vi "加标回收调试界面.vi"() -> ()   [LabVIEW 2016, in "质控单元V1.lvlib"]
uses:
  <vilib>/Utility/miscctls.llb/LVPointTypeDef.ctl
  <vilib>/Utility/miscctls.llb/LVPositionTypeDef.ctl
panel:
  in  "关闭":bool
  in  "请选择模块":T1(radio)=enum."氨氮"
  in  "关于":bool
  in  "Tab Control 4":enum32{"参数"}(tab)
  out "加标体积":string
  out "告警状态":string
  out "液位状态":string
  out "运行状态":string
  out "通讯状态":bool caption="状态"
  in  "Tab Control 3":enum32{"参数设置"}(tab)
  out "Y3":bool
  out "Y1":bool
  out "Y0":bool
  out "X1":bool
  out "X0":bool
  out "脉冲数":i32
  out "频率":i32
  in  "定时刷新":bool
  in  "流程参数读取":bool
  in  "流程参数写入":bool
  out "排液时间":sgl format="%.2f"
  out "搅拌时间":sgl format="%.2f"
  out "进样时间":sgl format="%.2f"
  out "润洗进样时间2":sgl format="%.2f"
  out "润洗排液时间2":sgl format="%.2f"
  out "润洗排液时间1":sgl format="%.2f"
  out "润洗进样时间1":sgl format="%.2f"
  in  "加标体积读取":bool
  in  "加标体积写入":bool
  in  "B":sgl
  in  "K":sgl
  in  "加标体积(mL)":sgl
  in  "注射泵系数读取":bool
  in  "注射泵系数写入":bool
  in  "Tab Control 2":enum32{"参数"}(tab)
  in  "启动水样润洗流程":bool
  in  "启动进样流程":bool
  in  "启动加标流程":bool
  in  "启动排液流程":bool
  in  "停止所有流程":bool
  in  "组合操作进水样":T2
  in  "清除告警":bool
  in  "启动搅拌流程":bool
  in  "加标":bool
  in  "注射泵注入量":sgl=0.1 min=0 max=1000 format="%#.6f mL"
  in  "组合操作排废液":T2
  in  "组合操作进空气":T2
  in  "组合操作慢速到液位":T2
  in  "组合操作进样调速":T2
  # "仪器状态"
  # "(默认30S)"
  # "柱塞泵泵系数"
  # "(默认50S)"
  # "(默认140S)"
  # "(默认500S)"
  # "(默认500S)"
  # "IO状态"
  # "(默认60S)"
  # "(默认140S)"
  # "组合步骤"
  # "测试流程"
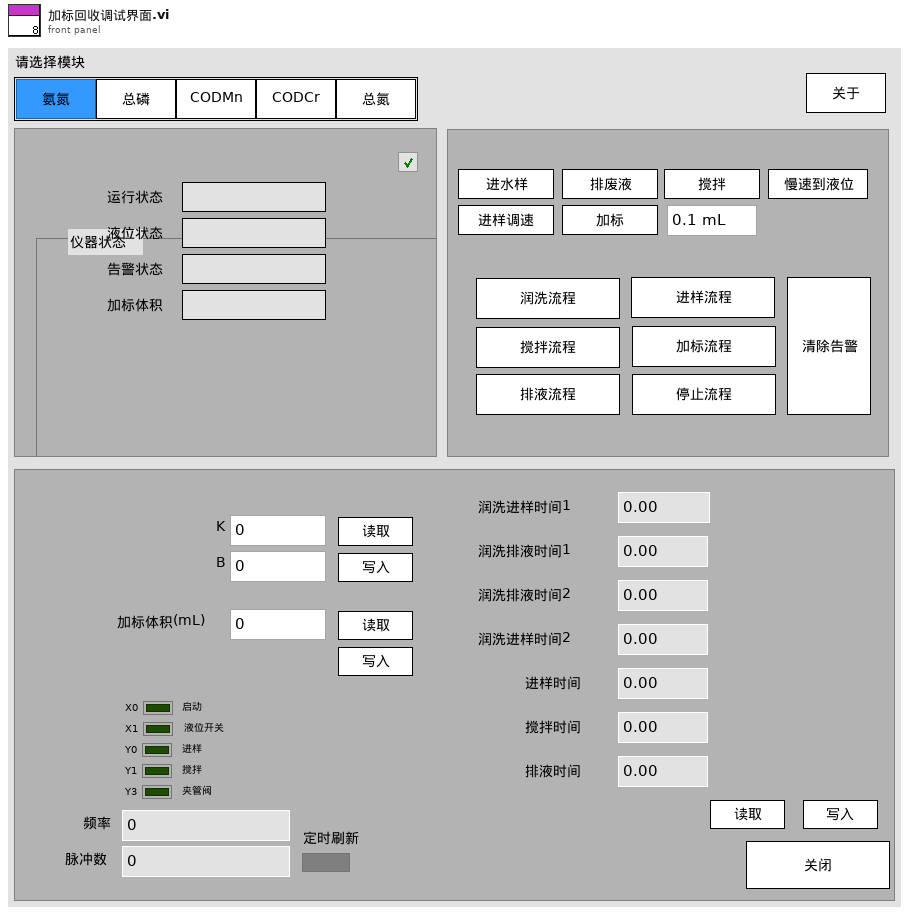
[diagram p1: front panel]
types:
  T1 = enum32{"未选择", "氨氮", "总磷", "CODMn", "CODCr", "总氮"}
  T2 = typedef "质控单元V1.lvlib/布尔控件.ctl" = bool
  T3 = typedef "LVPositionTypeDef.ctl" = cluster{"Left":i32, "Top":i32}
  T4 = typedef "LVPointTypeDef.ctl" = cluster{"Horizontal":i16, "Vertical":i16}
  T5 = typedef "质控单元V1.lvlib/质控slave id.ctl" = enum16{"null", "氨氮", "总磷", "CODMn", "CODCr", "总氮"}
  T6 = typedef "质控单元V1.lvlib/质控流程控制.ctl" = enum16{"待机", "润洗", "进样", "加标", "排液", "搅拌"}
  T7 = typedef "质控单元V1.lvlib/质控仪器状态显示.ctl" = cluster{"运行模式":string, "运行状态":string, "液位状态":string, "告警状态":string, "加标体积":string}
  T8 = cluster{"X0":bool, "X1":bool, "Y0":bool, "Y1":bool, "Y2":bool, "Y3":bool, "频率":i32, "脉冲数":i32}
  T9 = cluster{"润洗进样时间":sgl, "润洗排液时间1":sgl, "润洗排液时间2":sgl, "润洗超时时间":sgl, "进样超时时间":sgl, "搅拌时间":sgl, "排液时间":sgl}
  T10 = cluster{"润洗进样时间1":sgl, "润洗排液时间1":sgl, "润洗排液时间2":sgl, "润洗进样时间2":sgl, "进样时间":sgl, "搅拌时间":sgl, "排液时间":sgl}
  T11 = typedef "LVRectTypeDef.ctl" = cluster{"Left":i16, "Top":i16, "Right":i16, "Bottom":i16}
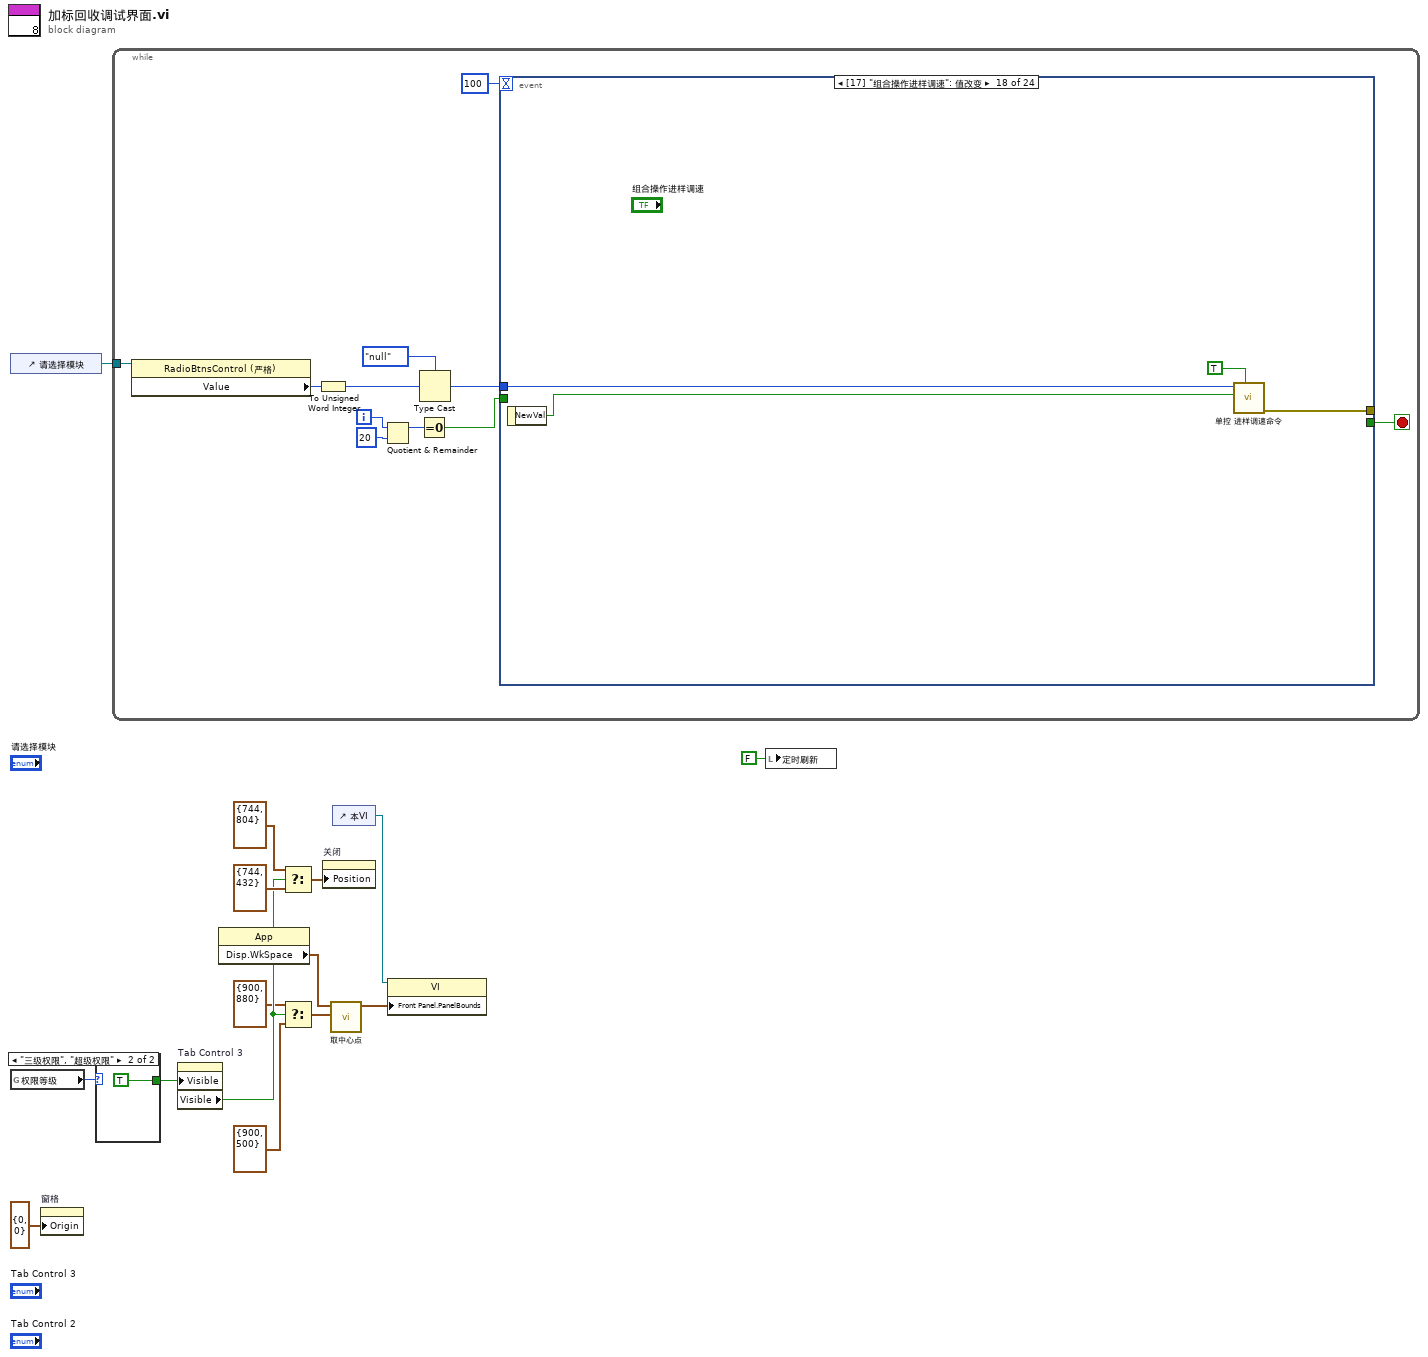
[diagram p0: block diagram]
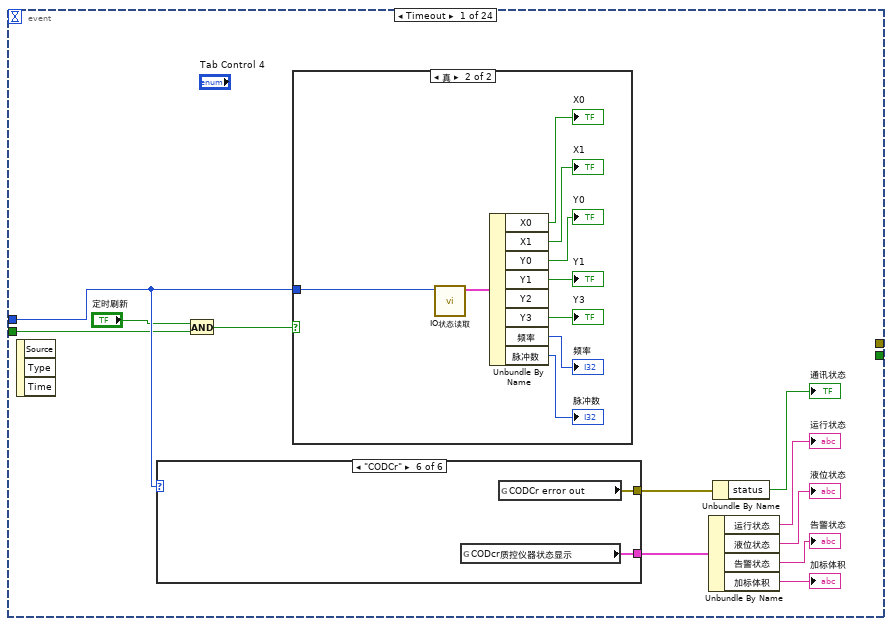
[diagram p3: hidden frame]
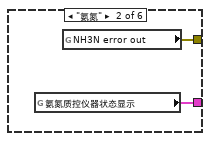
[diagram p6: hidden frame]
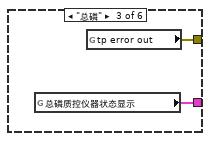
[diagram p7: hidden frame]
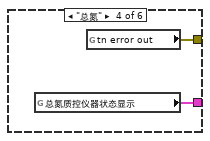
[diagram p8: hidden frame]
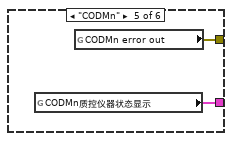
[diagram p9: hidden frame]
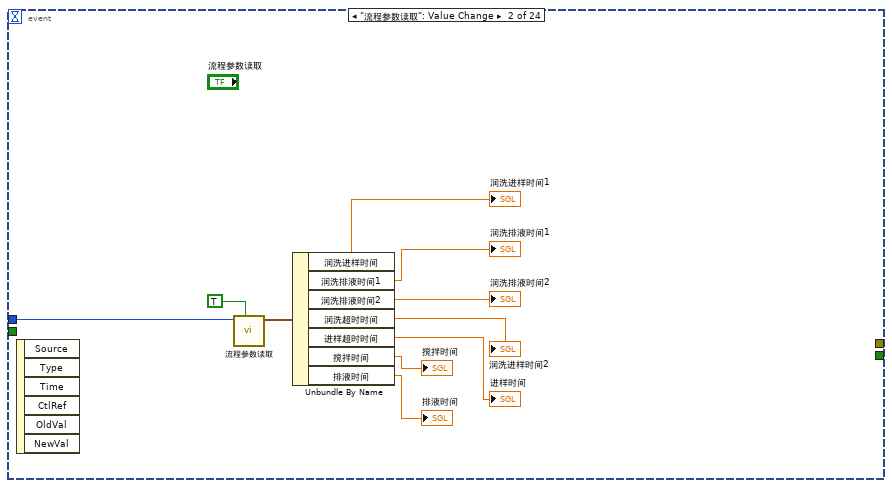
[diagram p10: hidden frame]
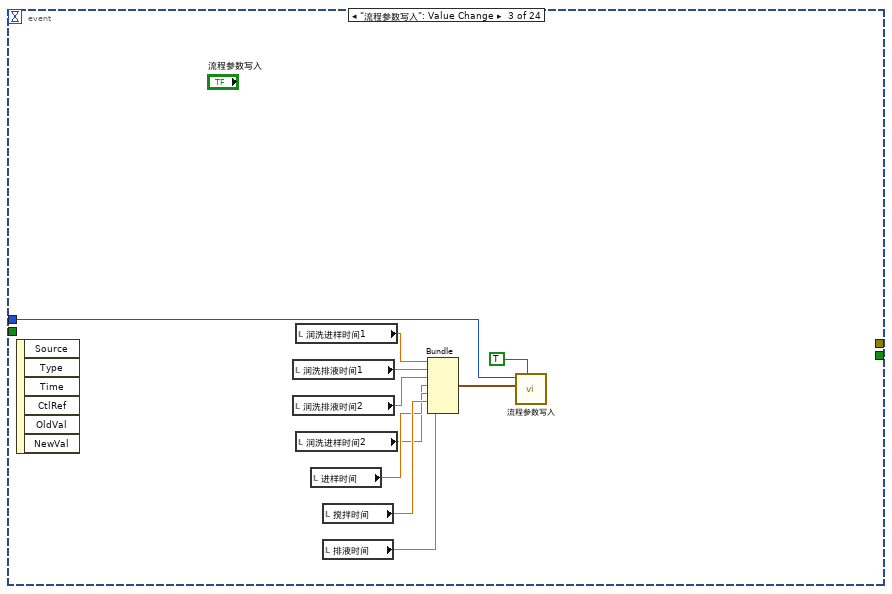
[diagram p11: hidden frame]
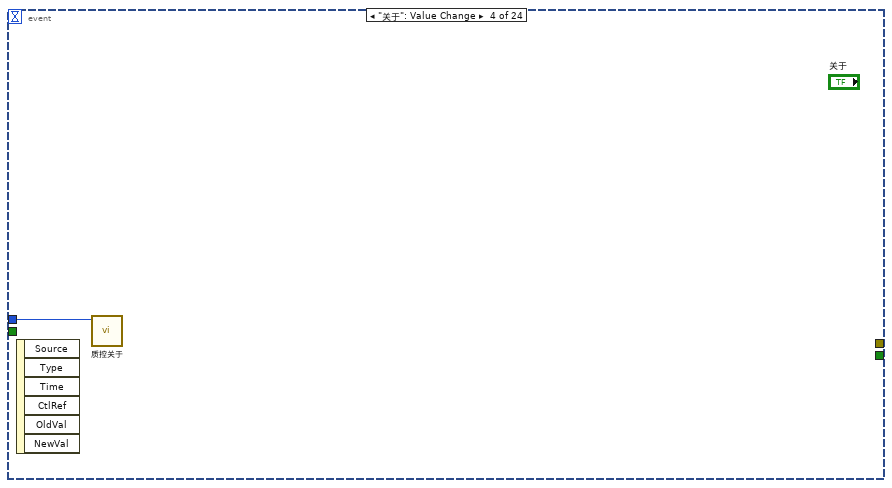
[diagram p12: hidden frame]
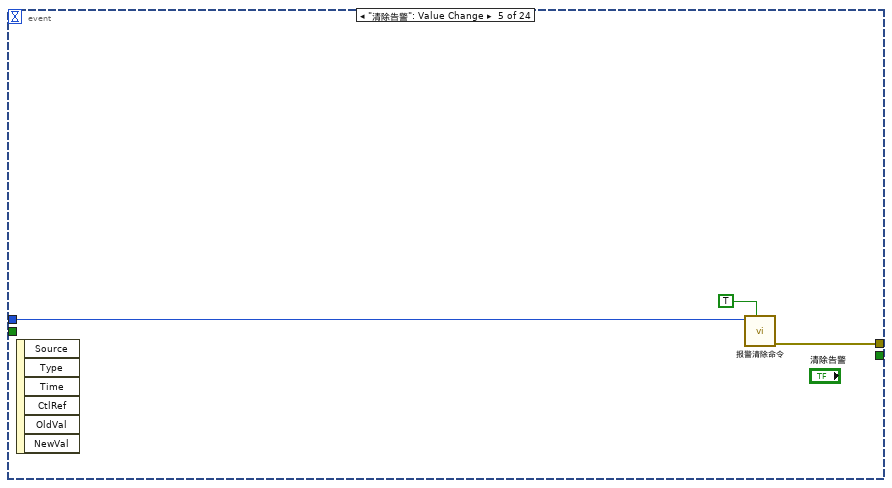
[diagram p13: hidden frame]
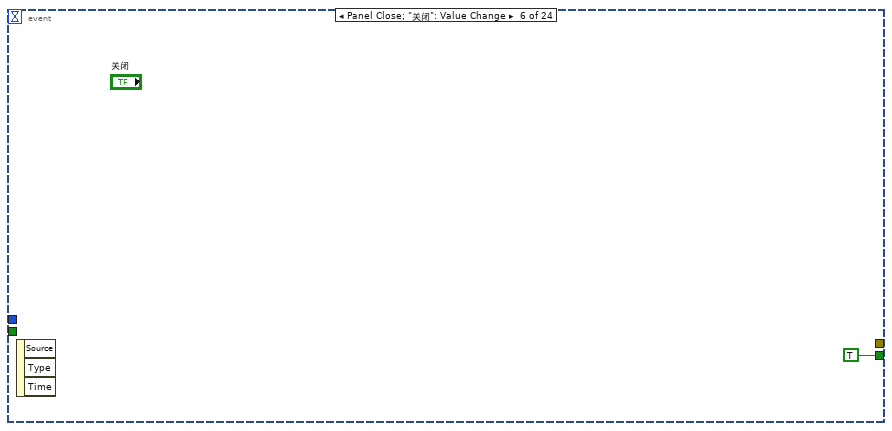
[diagram p14: hidden frame]
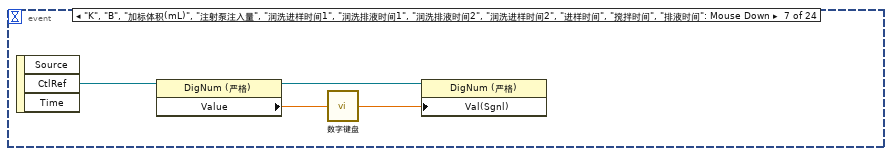
[diagram p15: hidden frame]
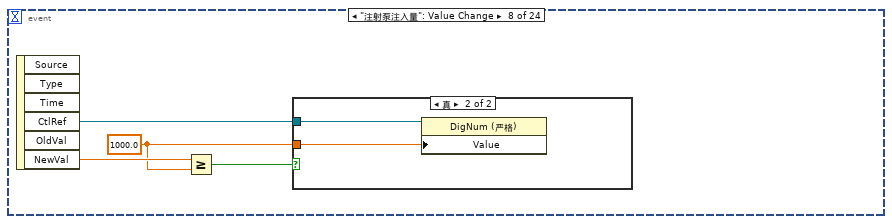
[diagram p16: hidden frame]
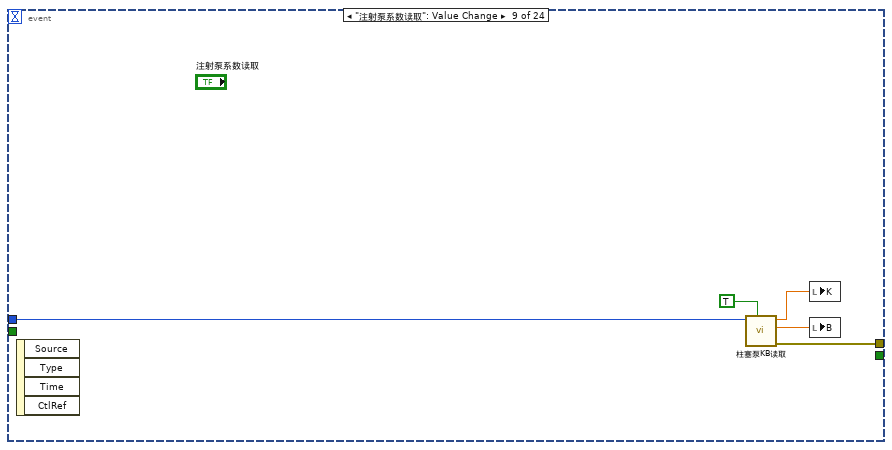
[diagram p18: hidden frame]
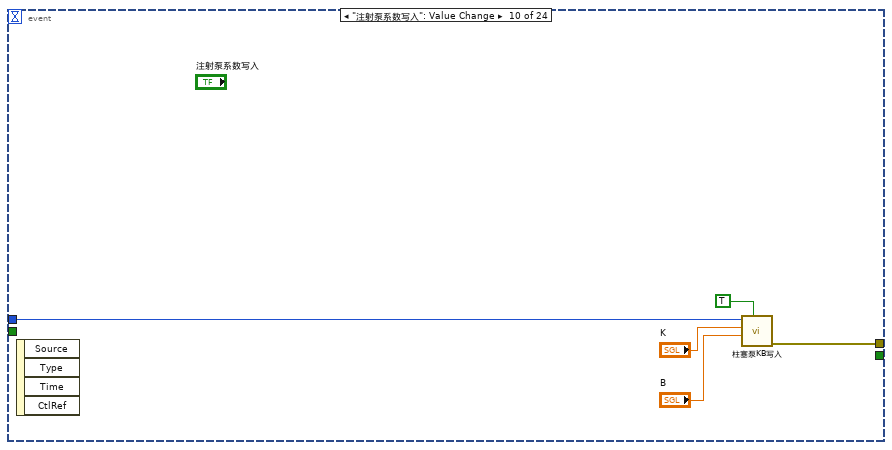
[diagram p19: hidden frame]
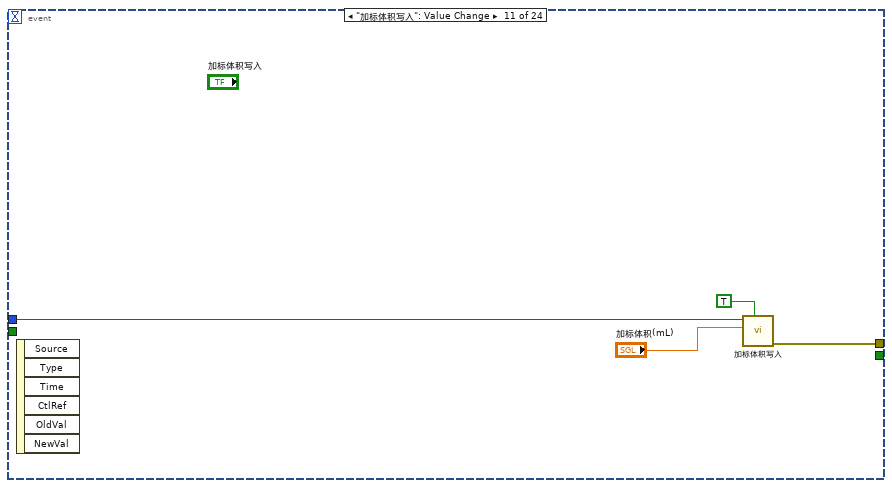
[diagram p20: hidden frame]
diagram:
  n1 = control-ref of="请选择模块"() -> (w14:refnum<vi>)
  n2 = global read "ZK非断电保存全局变量.vi" "权限等级"() -> (w3:enum16{"一级权限", "二级权限", "三级权限", "超级权限"})
  n3 = property on="窗格" class="Pane"("Origin"=T4 {"Horizontal"=0, "Vertical"=0} ("原点")) -> ()  [unwired: 2 in, 2 out]
  n4 = case shown="\"三级权限\", \"超级权限\"" w3 {
    tunnel: [_ TRUE] -> w2
    frame "一级权限", Default {
    }
    frame "三级权限", "超级权限" {
    }
  }
  n5 = while {
    tunnel: w14 -> [w25]
    i -> [w20]
    stop <- w27 stop-if-true
    n6 = property class="RadioBtnsControl (严格)"(reference=w25) -> ("Value"=w22:T1)  [unwired: 1 in, 2 out]
    n7 = To Unsigned Word Integer(number=w22) -> (unsigned 16bit integer=w21:u16)
    n8 = Quotient & Remainder(x=w20, y=20) -> (x-y*floor(x/y)=w18:i32)  [unwired: 1 out]
    n9 = Equal To 0?(x=w18) -> (x = 0?=w17:bool)
    n10 = Type Cast(type=质控slave_id."null" ("请选择模块"), x=w21) -> (*(type *) &x=w23:T5)
    n11 = event shown="[17] \"组合操作进样调速\": 值改变" {
      selector: _ -> [_ _ _ _ _ _ _ _ _ _ _ _ _ _ _ _ _ _ _ _ _ _ _ _]
      dyn-events: _ -> [_ _ _ _ _ _ _ _ _ _ _ _ _ _ _ _ _ _ _ _ _ _ _ _]
      timeout: 100 -> [_ _ _ _ _ _ _ _ _ _ _ _ _ _ _ _ _ _ _ _ _ _ _ _]
      tunnel: [_ _ _ _ _ TRUE _ _ _ _ _ _ _ _ _ _ _ _ _ _ _ _ _ _] -> w27
      tunnel: [_ _ _ _ w81 _ _ _ w95 w102 w106 w110 w113 w120 w124 w128 w132 w136 w140 w144 w148 w152 w155 w159] -> _
      tunnel: w23 -> [w31 w67 w77 w78 w79 _ _ _ w93 w100 w103 w107 w112 w118 w122 w126 w130 w134 w138 w141 w145 w149 w153 w157]
      tunnel: w17 -> [w29 _ _ _ _ _ _ _ _ _ _ _ _ _ _ _ _ _ _ _ _ _ _ _]
      event Timeout {
        n12 = event-data() -> ()  [unwired: 1 in, 3 out]
        n13 = case shown="\"CODCr\"" w31 {
          tunnel: [_ w49 w51 w53 w55 w57] -> w38
          tunnel: [_ w48 w50 w52 w54 w56] -> w33
          frame "null", Default {
          }
          frame "氨氮" {
            n14 = global read "ZK非断电保存全局变量.vi" "氨氮质控仪器状态显示"() -> (w49:T7)
            n15 = global read "ZK非断电保存全局变量.vi" "NH3N error out"() -> (w48:errorcluster)
          }
          frame "总磷" {
            n16 = global read "ZK非断电保存全局变量.vi" "总磷质控仪器状态显示"() -> (w51:T7)
            n17 = global read "ZK非断电保存全局变量.vi" "tp error out"() -> (w50:errorcluster)
          }
          frame "总氮" {
            n18 = global read "ZK非断电保存全局变量.vi" "总氮质控仪器状态显示"() -> (w53:T7)
            n19 = global read "ZK非断电保存全局变量.vi" "tn error out"() -> (w52:errorcluster)
          }
          frame "CODMn" {
            n20 = global read "ZK非断电保存全局变量.vi" "CODMn质控仪器状态显示"() -> (w55:T7)
            n21 = global read "ZK非断电保存全局变量.vi" "CODMn error out"() -> (w54:errorcluster)
          }
          frame "CODCr" {
            n22 = global read "ZK非断电保存全局变量.vi" "CODcr质控仪器状态显示"() -> (w57:T7)
            n23 = global read "ZK非断电保存全局变量.vi" "CODCr error out"() -> (w56:errorcluster)
          }
        }
        n24 = And(x="定时刷新", y=w29) -> (x .and. y?=w28:bool)
        n25 = case shown="真" w28 {
          tunnel: w31 -> [_ w47]
          frame False {
          }
          frame True {
            n26 = call "IO状态读取.vi"("Slave ID"=w47) -> ("STATES"=w46:T8)  [unwired: 9 in, 1 out]
            n27 = Unbundle By Name(w46) -> ("X0"=→"X0":bool, "X1"=→"X1":bool, "Y0"=→"Y0":bool, "Y1"=→"Y1":bool, "Y3"=→"Y3":bool, "频率"=→"频率":i32, "脉冲数"=→"脉冲数":i32)  [unwired: 1 out]
          }
        }
        n28 = Unbundle By Name(w38) -> ("运行状态"=→"运行状态":string, "液位状态"=→"液位状态":string, "告警状态"=→"告警状态":string, "加标体积"=→"加标体积":string)
        n29 = Unbundle By Name(w33) -> ("status"=→"通讯状态":bool)
      }
      event "流程参数读取": Value Change {
        n30 = event-data() -> ()  [unwired: 1 in, 6 out]
        n31 = call "流程参数读取.vi"("是否启用通讯通知"=TRUE, "Slave ID"=w67) -> ("参数"=w65:T9)  [unwired: 8 in, 1 out]
        n32 = Unbundle By Name(w65) -> ("润洗进样时间"=→"润洗进样时间1":sgl, "润洗排液时间1"=→"润洗排液时间1":sgl, "润洗排液时间2"=→"润洗排液时间2":sgl, "润洗超时时间"=→"润洗进样时间2":sgl, "进样超时时间"=→"进样时间":sgl, "搅拌时间"=→"搅拌时间":sgl, "排液时间"=→"排液时间":sgl)
      }
      event "流程参数写入": Value Change {
        n33 = event-data() -> ()  [unwired: 1 in, 6 out]
        n34 = local read "润洗排液时间1"() -> (w70:sgl)
        n35 = local read "润洗排液时间2"() -> (w71:sgl)
        n36 = local read "润洗进样时间1"() -> (w69:sgl)
        n37 = local read "润洗进样时间2"() -> (w72:sgl)
        n38 = local read "进样时间"() -> (w73:sgl)
        n39 = local read "搅拌时间"() -> (w74:sgl)
        n40 = local read "排液时间"() -> (w75:sgl)
        n41 = Bundle("润洗进样时间1"=w69, "润洗排液时间1"=w70, "润洗排液时间2"=w71, "润洗进样时间2"=w72, "进样时间"=w73, "搅拌时间"=w74, "排液时间"=w75) -> (w68:T10)  [unwired: 1 in]
        n42 = call "流程参数写入.vi"("是否启用通讯通知"=TRUE, "参数"=w68, "Slave ID"=w77) -> ()  [unwired: 8 in, 1 out]
      }
      event "关于": Value Change {
        n43 = event-data() -> ()  [unwired: 1 in, 6 out]
        n44 = call "质控关于.vi"("Slave ID"=w78) -> ()  [unwired: 11 in]
      }
      event "清除告警": Value Change {
        n45 = event-data() -> ()  [unwired: 1 in, 6 out]
        n46 = call "报警清除命令.vi"("是否启用通讯通知"=TRUE, "Slave ID"=w79) -> ("error out"=w81:errorcluster)  [unwired: 9 in]
      }
      event Panel Close; "关闭": Value Change {
        n47 = event-data() -> ()  [unwired: 1 in, 3 out]
      }
      event "K", "B", "加标体积(mL)", "注射泵注入量", "润洗进样时间1", "润洗排液时间1", "润洗排液时间2", "润洗进样时间2", "进样时间", "搅拌时间", "排液时间": Mouse Down {
        n48 = event-data() -> ("CtlRef"=w86:refnum<vi>)  [unwired: 1 in, 2 out]
        n49 = property class="DigNum (严格)"(reference=w86) -> (reference out=w85:refnum<vi>, "Value"=w83:sgl)  [unwired: 1 in, 1 out]
        n50 = call "数字键盘.vi"("OldNumber"=w83) -> ("NewNumber"=w84:sgl)
        n51 = property class="DigNum (严格)"(reference=w85, "Val(Sgnl)"=w84) -> ()  [unwired: 1 in, 2 out]
      }
      event "注射泵注入量": Value Change {
        w88 = sgl 1000.0 ("y")
        n52 = event-data() -> ("CtlRef"=w89:refnum<vi>, "NewVal"=w90:sgl)  [unwired: 1 in, 4 out]
        n53 = Greater Or Equal?(x=w90, y=w88) -> (x >= y?=w87:bool)
        n54 = case shown="真" w87 {
          tunnel: w89 -> [_ w92]
          tunnel: w88 -> [_ w91]
          frame False {
          }
          frame True {
            n55 = property class="DigNum (严格)"(reference=w92, "Value"=w91) -> ()  [unwired: 1 in, 2 out]
          }
        }
      }
      event "注射泵系数读取": Value Change {
        n56 = event-data() -> ()  [unwired: 1 in, 4 out]
        n57 = call "柱塞泵KB读取.vi"("是否启用通讯通知"=TRUE, "Slave ID"=w93) -> ("error out"=w95:errorcluster, "B"=w96:sgl, "K"=w97:sgl)  [unwired: 7 in]
        n58 = local write "K"(w97) -> ()
        n59 = local write "B"(w96) -> ()
      }
      event "注射泵系数写入": Value Change {
        n60 = event-data() -> ()  [unwired: 1 in, 4 out]
        n61 = call "柱塞泵KB写入.vi"("是否启用通讯通知"=TRUE, "B"="B", "K"="K", "Slave ID"=w100) -> ("error out"=w102:errorcluster)  [unwired: 7 in]
      }
      event "加标体积写入": Value Change {
        n62 = event-data() -> ()  [unwired: 1 in, 6 out]
        n63 = call "加标体积写入.vi"("是否启用通讯通知"=TRUE, "加标体积"="加标体积(mL)", "Slave ID"=w103) -> ("error out"=w106:errorcluster)  [unwired: 8 in]
      }
      event "加标体积读取": Value Change {
        n64 = event-data() -> ()  [unwired: 1 in, 6 out]
        n65 = call "加标体积读取.vi"("是否启用通讯通知"=TRUE, "Slave ID"=w107) -> ("error out"=w110:errorcluster, "加标体积"=w109:sgl)  [unwired: 8 in]
        n66 = local write "加标体积(mL)"(w109) -> ()
      }
      event "加标": Value Change {
        n67 = event-data() -> ()  [unwired: 1 in, 6 out]
        n68 = call "加标体积写入.vi"("是否启用通讯通知"=FALSE, "加标体积"="注射泵注入量", "Slave ID"=w112) -> ("error out"=w114:errorcluster)  [unwired: 8 in]
        n69 = call "单控 柱塞泵命令.vi"("是否启用通讯通知"=TRUE, "error in (no error)"=w114, "Slave ID"=w112) -> ("error out"=w113:errorcluster)  [unwired: 8 in]
      }
      event Value Change {
        n70 = event-data() -> ("NewVal"=w117:T2)  [unwired: 1 in]
        n71 = call "单控 进样命令.vi"("是否启用通讯通知"=TRUE, "进样"=w117, "Slave ID"=w118) -> ("error out"=w120:errorcluster)  [unwired: 8 in]
      }
      event Value Change {
        n72 = event-data() -> ("NewVal"=w121:T2)  [unwired: 1 in]
        n73 = call "单控 排液命令.vi"("是否启用通讯通知"=TRUE, "排液"=w121, "Slave ID"=w122) -> ("error out"=w124:errorcluster)  [unwired: 8 in]
      }
      event Value Change {
        n74 = event-data() -> ("NewVal"=w125:T2)  [unwired: 1 in]
        n75 = call "单控 搅拌命令.vi"("是否启用通讯通知"=TRUE, "搅拌"=w125, "Slave ID"=w126) -> ("error out"=w128:errorcluster)  [unwired: 8 in]
      }
      event Value Change {
        n76 = event-data() -> ("NewVal"=w129:T2)  [unwired: 1 in]
        n77 = call "单控 慢速到液位命令.vi"("是否启用通讯通知"=TRUE, "慢速到液位"=w129, "Slave ID"=w130) -> ("error out"=w132:errorcluster)  [unwired: 8 in]
      }
      event Value Change {
        n78 = event-data() -> ("NewVal"=w133:T2)  [unwired: 1 in]
        n79 = call "单控 进样调速命令.vi"("是否启用通讯通知"=TRUE, "进样调速"=w133, "Slave ID"=w134) -> ("error out"=w136:errorcluster)  [unwired: 8 in]
      }
      event "启动进样流程": Value Change {
        n80 = event-data() -> ()  [unwired: 1 in, 6 out]
        n81 = call "单步流程命令.vi"("是否启用通讯通知"=TRUE, "流程控制"=质控流程控制."进样", "Slave ID"=w138) -> ("error out"=w140:errorcluster)  [unwired: 8 in]
      }
      event "启动加标流程": Value Change {
        n82 = event-data() -> ()  [unwired: 1 in, 6 out]
        n83 = call "单步流程命令.vi"("是否启用通讯通知"=TRUE, "流程控制"=质控流程控制."加标", "Slave ID"=w141) -> ("error out"=w144:errorcluster)  [unwired: 8 in]
      }
      event "启动排液流程": Value Change {
        n84 = event-data() -> ()  [unwired: 1 in, 6 out]
        n85 = call "单步流程命令.vi"("是否启用通讯通知"=TRUE, "流程控制"=质控流程控制."排液", "Slave ID"=w145) -> ("error out"=w148:errorcluster)  [unwired: 8 in]
      }
      event "启动搅拌流程": Value Change {
        n86 = event-data() -> ()  [unwired: 1 in, 6 out]
        n87 = call "单步流程命令.vi"("是否启用通讯通知"=TRUE, "流程控制"=质控流程控制."搅拌", "Slave ID"=w149) -> ("error out"=w152:errorcluster)  [unwired: 8 in]
      }
      event "停止所有流程": Value Change {
        n88 = event-data() -> ()  [unwired: 1 in, 6 out]
        n89 = call "停止命令.vi"("是否启用通讯通知"=TRUE, "Slave ID"=w153) -> ("error out"=w155:errorcluster)  [unwired: 9 in]
      }
      event "启动水样润洗流程": Value Change {
        n90 = event-data() -> ()  [unwired: 1 in, 6 out]
        n91 = call "单步流程命令.vi"("是否启用通讯通知"=TRUE, "流程控制"=质控流程控制."润洗", "Slave ID"=w157) -> ("error out"=w159:errorcluster)  [unwired: 8 in]
      }
    }
  }
  n92 = property on="Tab Control 3" class="TabCtl (严格)"("Visible"=w2) -> ("Visible"=w9:bool)  [unwired: 2 in, 2 out]
  n93 = property class="App"() -> ("Disp.WkSpace"=w7:T11)  [unwired: 2 in, 2 out]
  n94 = Select(t=T3 {"Left"=744, "Top"=804} ("位置"), s=w9, f=T3 {"Left"=744, "Top"=432} ("位置")) -> (s? t:f=w11:T3)
  n95 = Select(t=T3 {"Left"=900, "Top"=880} ("位置"), s=w9, f=T3 {"Left"=900, "Top"=500} ("位置")) -> (s? t:f=w6:T3)
  n96 = property on="关闭" class="Bool"("Position"=w11) -> ()  [unwired: 2 in, 2 out]
  n97 = call "取中心点.vi"("前面板窗口:最小尺寸"=w6, "显示:主工作区"=w7) -> ("前面板窗口:窗口边界"=w5:T11)  [unwired: 9 in]
  n98 = control-ref of="本VI"() -> (w4:refnum<vi>)
  n99 = property class="VI"(reference=w4, "Front Panel.PanelBounds"=w5) -> ()  [unwired: 1 in, 2 out]
  n100 = local write "定时刷新"(FALSE ("定时刷新")) -> ()
